vi "Auton_S2_Right_Switch.vi"   [LabVIEW 2017]
uses:
  <vilib>/Rock Robotics/WPI/Utilities/WPI_GetSetVariantRefNum.vi
  Robot Global Data.vi
  <vilib>/Rock Robotics/WPI/RobotDrive/WPI_RobotDriveArcadeDrive_Standard(NoSaturation).vi
types:
  T1 = typedef "WPI_RobotDriveDevRef.ctl" = cluster{"DevStatus":errorcluster, "Motors[]":T2[], "Square Inputs":bool, "Max Output":dbl}
  T2 = typedef "WPI_MotorControlDeviceRef.ctl" = cluster{"DeviceStatus":errorcluster, "Type":T3, "PWM":cluster{"PWM Channel":T4, "DeadBand":T5}, "CAN":cluster{"Device Number":u8, "SetOutput VI Ref":variant, "GetOutput VI Ref":variant, "Enable VI Ref":variant, "Disable VI Ref":variant, "Data":variant}, "Invert":bool, "DIO PWM":cluster{"PWM \"Enable\" Channel":T4, "DIOChannel":T6, "PWM Rate":dbl}}
  T3 = typedef "WPI_MotorControlType.ctl" = enum16{"PWM", "CAN", "DIO PWM"}
  T4 = typedef "FPGA_DIOPWMChannel.ctl" = enum8{"PWM 0", "PWM 1", "PWM 2", "PWM 3", "PWM 4", "PWM 5", "PWM 6", "PWM 7", "PWM 8", "PWM 9", "PWM MXP 0", "PWM MXP 1", "PWM MXP 2", "PWM MXP 3", "PWM MXP 4", "PWM MXP 5", "PWM MXP 6", "PWM MXP 7", "PWM MXP 8", "PWM MXP 9", "Invalid"}
  T5 = typedef "WPI_PWMDeadband.ctl" = cluster{"Name":string, "maxPositivePwm":i32, "minPositivePwm":i32, "centerPwm":i32, "maxNegativePwm":i32, "minNegativePwm":i32, "angularRange":u16}
  T6 = typedef "FPGA_DIOChannel.ctl" = enum8{"DIO 0", "DIO 1", "DIO 2", "DIO 3", "DIO 4", "DIO 5", "DIO 6", "DIO 7", "DIO 8", "DIO 9", "DIO MXP 0", "DIO MXP 1", "DIO MXP 2", "DIO MXP 3", "DIO MXP 4", "DIO MXP 5", "DIO MXP 6", "DIO MXP 7", "DIO MXP 8", "DIO MXP 9", "DIO MXP 10", "DIO MXP 11", "DIO MXP 12", "DIO MXP 13", "DIO MXP 14", "DIO MXP 15", "SPI Port CS1", "SPI Port CS2", "SPI Port CS3", "SPI Port MISO", "SPI Port MOSI", "Invalid"}
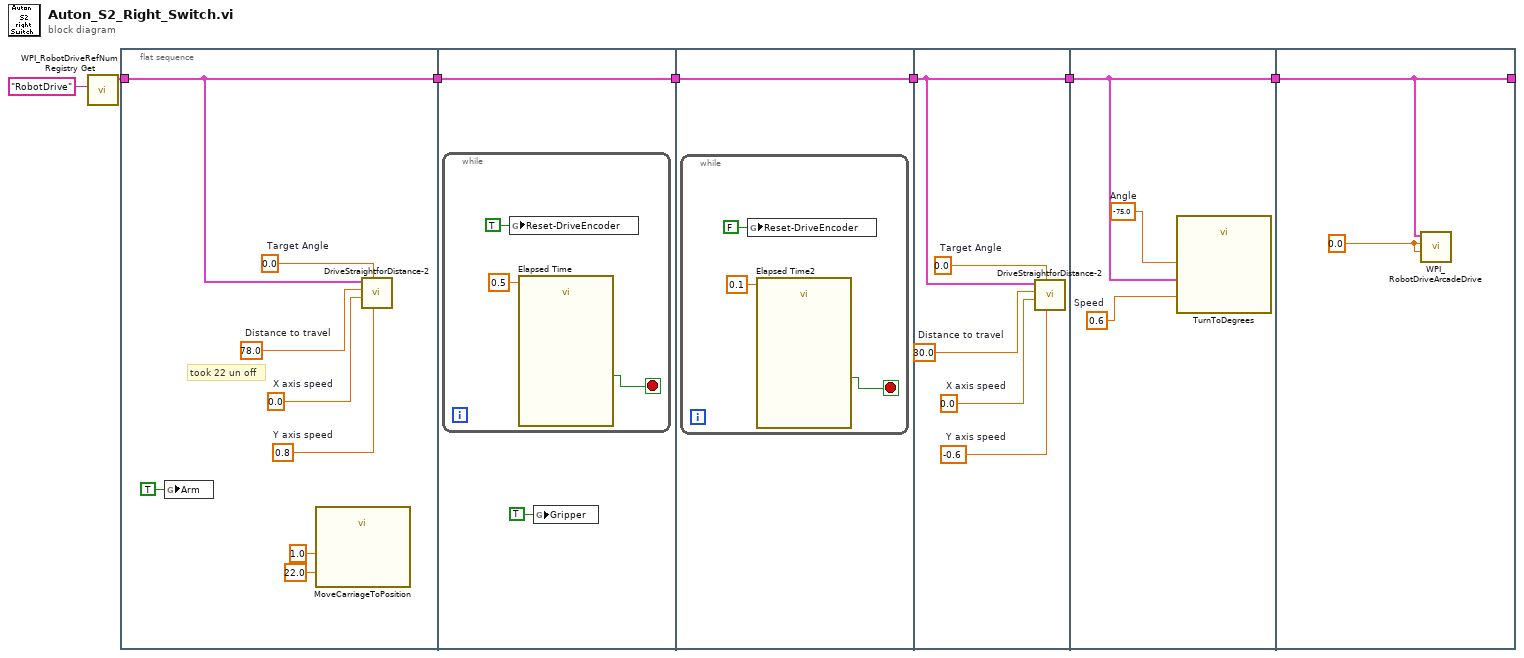
[diagram p0: block diagram]
diagram:
  n1 = call <vilib>:"WPI_RobotDriveRefNum Registry Get.vi"("refnum name"="RobotDrive") -> ("RobotDriveDevRef"=w6:T1)  [unwired: 9 in, 1 out]
  n2 = flat-sequence {
    tunnel: [w15] -> w5
    tunnel: w6 -> [w15]
    tunnel: w5 -> [w17]
    tunnel: [w17] -> w4
    tunnel: w4 -> [w21]
    tunnel: [w21] -> w3
    tunnel: w3 -> [w25]
    tunnel: [w25] -> w2
    tunnel: w2 -> [w30]
    tunnel: [w30] -> w1
    tunnel: [w33] -> _
    tunnel: w1 -> [w33]
    frame #0 {
      w11 = 0.0  # Target Angle
      w12 = 0.8  # Y axis speed
      w13 = 0.0  # X axis speed
      w14 = 78.0  # Distance to travel
      # "took 22 un off"
      n3 = global write "Robot Global Data.vi" "Arm"(TRUE ("Arm")) -> ()
      n4 = call "MoveCarriageToPosition.vi"("Lift Speed"=1.0, "Target Height"=22.0) -> ()  [unwired: 10 in]
      n5 = call "DriveStraightforDistance-2.vi"("Y axis speed"=w12, "Target Angle"=w11, "X axis speed"=w13, "Distance to travel"=w14, "RobotDriveDevRef"=w15) -> ()  [unwired: 7 in]
    }
    frame #1 {
      n6 = while {
        stop <- w20 stop-if-true
        n7 = global write "Robot Global Data.vi" "Reset-DriveEncoder"(TRUE ("Reset-DriveEncoder")) -> ()
        n8 = call "Elapsed Time"("Time Target (s)"=0.5) -> ("Time has Elapsed"=w20:bool)  [unwired: 11 in, 7 out]
      }
      n9 = global write "Robot Global Data.vi" "Gripper"(TRUE ("Gripper")) -> ()
    }
    frame #2 {
      n10 = while {
        stop <- w24 stop-if-true
        n11 = global write "Robot Global Data.vi" "Reset-DriveEncoder"(FALSE ("Reset-DriveEncoder")) -> ()
        n12 = call "Elapsed Time2"("Time Target (s)"=0.1) -> ("Time has Elapsed"=w24:bool)  [unwired: 11 in, 7 out]
      }
    }
    frame #3 {
      w26 = 0.0  # Target Angle
      w27 = -0.6  # Y axis speed
      w28 = 0.0  # X axis speed
      w29 = 30.0  # Distance to travel
      n13 = call "DriveStraightforDistance-2.vi"("Y axis speed"=w27, "Target Angle"=w26, "X axis speed"=w28, "Distance to travel"=w29, "RobotDriveDevRef"=w25) -> ()  [unwired: 7 in]
    }
    frame #4 {
      w31 = -75.0  # Angle
      w32 = 0.6  # Speed
      n14 = call "TurnToDegrees.vi"("Speed"=w32, "RobotDriveDevRef"=w30, "Angle"=w31) -> ()  [unwired: 9 in]
    }
    frame #5 {
      w34 = 0.0 ("X axis value")
      n15 = call-poly <vilib>:"WPI_RobotDriveArcadeDrive.vi"("Y axis value"=w34, "X axis value"=w34, "RobotDriveDevRef"=w33) -> ()  [unwired: 6 in, 3 out]
    }
  }
